vi "moveNext.vi"(8 "error in (no error)":errorcluster, 11 "IIterator in":refnum<class "IIterator.lvclass">) -> (0 "error out":errorcluster, 2 "errorCode out":T1 items=["OPENDAQ_SUCCESS"=0, "OPENDAQ_NO_MORE_ITEMS"=5], 3 "IIterator out":refnum<class "IIterator.lvclass">)   [LabVIEW 2022 SP3, in "openDAQ.lvlib" / "IBaseObject.lvlib" / "IIterator.lvlib" / "IIterator.lvclass"]
uses:
  <instrlib>/openDAQ/Public/Classes/IIterator/IIterator.lvclass
  C:/Program Files (x86)/National Instruments/LabVIEW 2022/instr.lib/openDAQ/Public/Classes/IBaseObject/IBaseObject.lvclass
  <instrlib>/openDAQ/Public/Classes/daqCoreTypes/Errors/TypeDef/errorCodes.ctl
  <instrlib>/openDAQ/Public/Classes/IBaseObject/IBaseObject.lvclass/IBaseObject.ctl
  <instrlib>/openDAQ/Public/Classes/IBaseObject/Accessor/Read reference.vi
  <instrlib>/openDAQ/Public/Classes/IBaseObject/Accessor/Write reference.vi
  <instrlib>/openDAQ/Binaries/Windows/x86/copendaq32.dll
  <instrlib>/openDAQ/Public/Classes/daqCoreTypes/Errors/Errors.lvclass
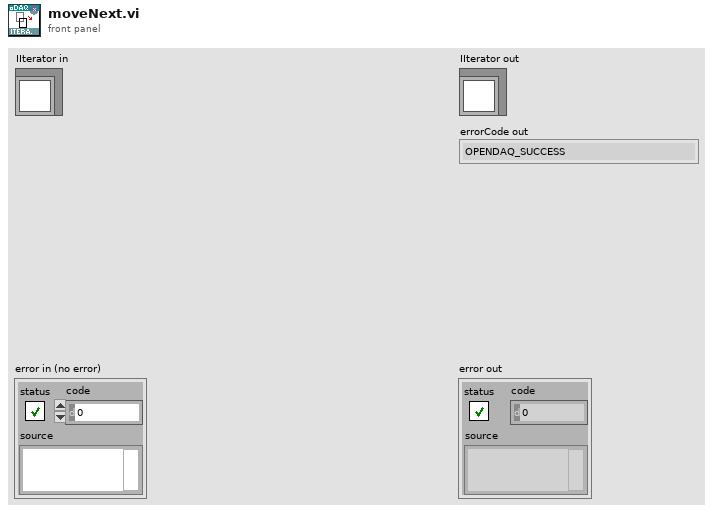
[diagram p1: front panel]
types:
  T1 = typedef "openDAQ.lvlib/daqCoreTypes.lvlib/Errors.lvclass/errorCodes.ctl" = u16
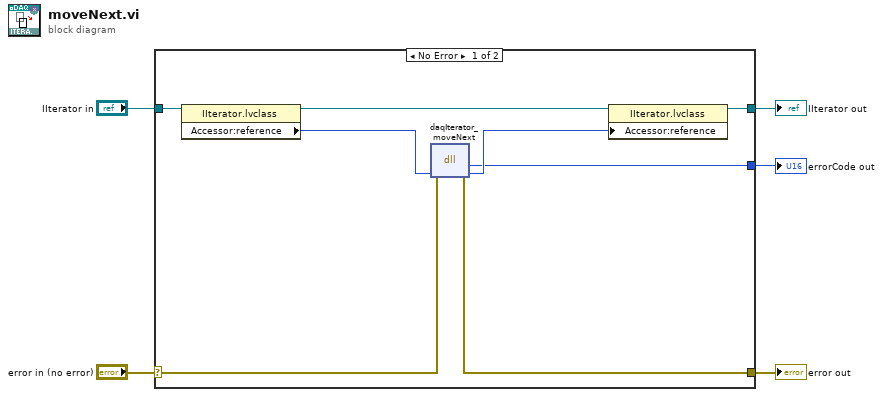
[diagram p0: block diagram]
diagram:
  n1 = case shown="No Error" "error in (no error)" {
    selector: "error in (no error)" -> [w8 w15]
    tunnel: [w7 w15] -> w4
    tunnel: [w11 w14] -> w2
    tunnel: "IIterator in" -> [w13 w14]
    tunnel: [w6 _] -> w1
    frame No Error {
      n2 = property class="IIterator.lvclass"(reference=w13) -> (reference out=w12:refnum<class "IIterator.lvclass">, "Accessor:reference"=w10:i64)  [unwired: 1 in, 1 out]
      n3 = dll-call lib="C:/Program Files (x86)/National Instruments/LabVIEW 2022/instr.lib/openDAQ/Binaries/Windows/x86/copendaq*.*" fn="daqIterator_moveNext"(error in=w8, "iterator"=w10) -> (error out=w7:errorcluster, "return type"=w6:u32, "iterator"=w9:i64)  [unwired: 2 in, 1 out]
      n4 = property class="IIterator.lvclass"(reference=w12, "Accessor:reference"=w9) -> (reference out=w11:refnum<class "IIterator.lvclass">)  [unwired: 1 in, 1 out]
    }
    frame Error {
    }
  }
  "error out" <- w4
  "IIterator out" <- w2
  "errorCode out" <- w1
